vi "Initialize.vi"(8 "error in":errorcluster, 9 "Slot Settings":T1, 11 "9253 in":refnum<class "9253.lvclass">) -> (0 "error out":errorcluster, 3 "9253 out":refnum<class "9253.lvclass">)   [LabVIEW 2017, in "Modules.lvlib" / "9253.lvclass"]
uses:
  9253.lvclass
  RSI Module/Slot Settings.ctl
  C:/Users/nitest/Documents/NI/niveristand-scan-engine-module-libraries/Source/RSI Module/RSI Module.lvclass
  RSI Module/Channels.ctl
  RSI Module/Channel Type.ctl
  RSI Module/Module Models.ctl
  9253.lvclass/9253.ctl
  RSI Module/RSI Module.lvclass
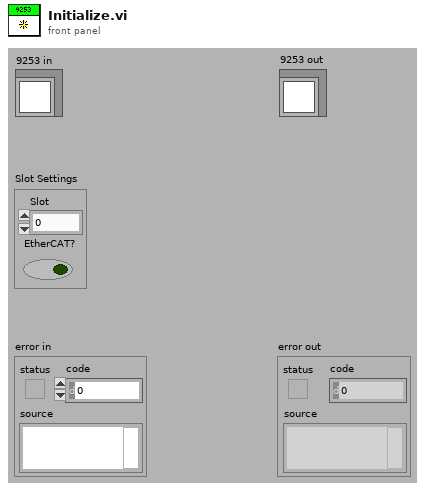
[diagram p1: front panel]
types:
  T1 = typedef "Modules.lvlib/RSI Module.lvclass/Slot Settings.ctl" = cluster{"Slot":u32, "EtherCAT?":bool}
  T2 = typedef "Modules.lvlib/RSI Module.lvclass/Channels.ctl" = cluster{"# Input Channels":i32, "# Output Channels":i32, "Channel Type":T3, "Units":string}
  T3 = typedef "Modules.lvlib/RSI Module.lvclass/Channel Type.ctl" = enum16{"Analog", "Digital"}
  T4 = typedef "Modules.lvlib/RSI Module.lvclass/Module Models.ctl" = enum16{"Empty", "NI 9201", "NI 9203", "NI 9205", "NI 9206", "NI 9207", "NI 9208", "NI 9209", "NI 9210", "NI 9211", "NI 9212", "NI 9213", "NI 9214", "NI 9215", "NI 9216", "NI 9217", "NI 9219", "NI 9220", "NI 9221", "NI 9222", "NI 9223", "NI 9224", "NI 9225", "NI 9226", "NI 9227", "NI 9228", "NI 9229", "NI 9233", "NI 9234", "NI 9235", "NI 9236", "NI 9237", "NI 9239", "NI 9242", "NI 9244", "NI 9253", "NI 9263", "NI 9264", "NI 9265", "NI 9266", "NI 9269", "NI 9344", "NI 9350", "NI 9375", "NI 9401", "NI 9402", "NI 9403", "NI 9411", "NI 9421", "NI 9422", "NI 9423", "NI 9425", "NI 9426", "NI 9435", "NI 9436", "NI 9437", "NI 9472", "NI 9474", "NI 9475", "NI 9476", "NI 9477", "NI 9478", "NI 9481", "NI 9482", "NI 9485"}
  T5 = cluster{"fault detection enable":bool, "lower fault detection limit":dbl, "upper fault detection limit":dbl}
  T6 = cluster{"fault detection enable":bool, "lower fault detection limit":dbl, "upper fault detection limit":dbl}[]
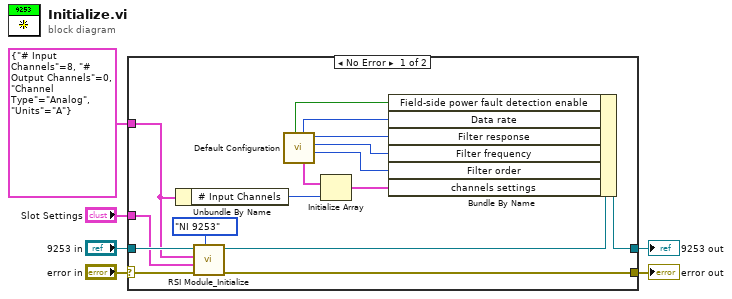
[diagram p0: block diagram]
diagram:
  n1 = case shown="No Error" "error in" {
    selector: "error in" -> [w20 w24]
    tunnel: [w17 w24] -> w5
    tunnel: [w18 w23] -> w3
    tunnel: "9253 in" -> [w22 w23]
    tunnel: "Slot Settings" -> [w21 _]
    tunnel: T2 {"# Input Channels"=8, "# Output Channels"=0, "Channel Type"=enum."Analog", "Units"="A"} ("Channels") -> [w15 _]
    frame No Error {
      n2 = Unbundle By Name(w15) -> ("# Input Channels"=w14:i32)
      n3 = call "RSI Module_Initialize.vi"("Module Model"=Module_Models."NI 9253", "error in (no error)"=w20, "Slot Settings"=w21, "Channels"=w15, "RSI Module in"=w22) -> ("error out"=w17:errorcluster, "RSI Module out"=w19:refnum<class "9253.lvclass">)  [unwired: 5 in]
      n4 = call "Default Configuration.vi"() -> ("Filter order"=w9:u32, "Filter frequency"=w10:u32, "Filter response"=w11:u32, "channel settings"=w12:T5, "Data rate"=w8:u32, "Field-side power fault detection enable"=w7:bool)  [unwired: 6 in]
      n5 = Initialize Array(w12, w14) -> (w13:T6)
      n6 = Bundle By Name(cluster=w19, "Field-side power fault detection enable"=w7, "Data rate"=w8, "Filter response"=w11, "Filter frequency"=w10, "Filter order"=w9, "channels settings"=w13) -> (w18:refnum<class "9253.lvclass">)
    }
    frame Error {
    }
  }
  "error out" <- w5
  "9253 out" <- w3
